vi "Serialization Test.vi"() -> ()   [LabVIEW 2017, in "GPIC Core tests.lvlib"]
uses:
  GPIC Core tests.lvlib
  module/configuration/GPIC Core configuration.lvclass
  module/configuration/GPIC Core configuration.lvclass/GPIC Core configuration.ctl
  <vilib>/NI/Tag Bus Module Framework/channel/TBM channel.lvclass
panel:
  out "lines equal 2":bool
  out "lines equal":bool
  out "modules equal":bool
  out "channels equal":bool
  out "no error":errorcluster
  out "no error 2":errorcluster
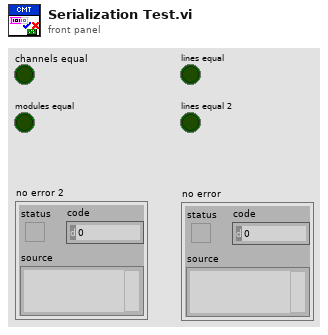
[diagram p1: front panel]
types:
  T1 = cluster{"channel":refnum<class "TBM channel.lvclass">}[]
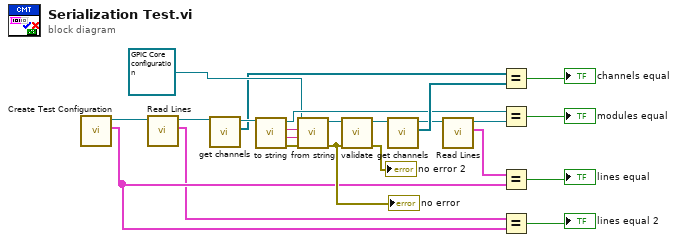
[diagram p0: block diagram]
diagram:
  n1 = call "Create Test Configuration.vi"() -> ("Line Array"=w5:T1, "Module"=w23:refnum<class "GPIC Core configuration.lvclass">)  [unwired: 6 in, 4 out]
  n2 = call "Read Lines.vi"("GPIC Core configuration in"=w23) -> ("Lines"=w4:T1, "GPIC Core configuration out"=w22:refnum<class "GPIC Core configuration.lvclass">)  [unwired: 8 in, 1 out]
  n3 = call-dynamic "get channels.vi"("fixed channel configuration in"=w22) -> ("channels"=w1:refnum<class "TBM channel.lvclass">[], "fixed channel configuration out"=w8:refnum<class "GPIC Core configuration.lvclass">)  [unwired: 9 in]
  n4 = call-dynamic "to string.vi"("fixed channel configuration in"=w8) -> ("error out"=w21:errorcluster, "data"=w20:string, "version"=w19:string, "fixed channel configuration out"=w11:refnum<class "GPIC Core configuration.lvclass">)  [unwired: 7 in]
  n5 = call-dynamic "from string.vi"("error in"=w21, "data"=w20, "version"=w19, "fixed channel configuration in"=refnum<class "GPIC Core configuration.lvclass"> refnum ("user control module configuration out")) -> ("error out"=w16:errorcluster, "fixed channel configuration out"=w18:refnum<class "GPIC Core configuration.lvclass">)  [unwired: 6 in]
  "no error" <- w16
  n6 = call-dynamic "validate.vi"("error in"=w16, "fixed channel configuration in"=w18) -> ("error out"=→"no error 2":errorcluster, "fixed channel configuration out"=w14:refnum<class "GPIC Core configuration.lvclass">)  [unwired: 8 in]
  n7 = call-dynamic "get channels.vi"("fixed channel configuration in"=w14) -> ("channels"=w13:refnum<class "TBM channel.lvclass">[], "fixed channel configuration out"=w6:refnum<class "GPIC Core configuration.lvclass">)  [unwired: 9 in]
  n8 = call "Read Lines.vi"("GPIC Core configuration in"=w6) -> ("Lines"=w3:T1, "GPIC Core configuration out"=w2:refnum<class "GPIC Core configuration.lvclass">)  [unwired: 8 in, 1 out]
  n9 = Equal?(x=w1, y=w13) -> (x = y?=→"channels equal":bool)
  n10 = Equal?(x=w11, y=w2) -> (x = y?=→"modules equal":bool)
  n11 = Equal?(x=w3, y=w5) -> (x = y?=→"lines equal":bool)
  n12 = Equal?(x=w4, y=w5) -> (x = y?=→"lines equal 2":bool)
